vi "SRDG535.panel.vi"(0 "object ref":refnum<vi>, 5 "error in (no error)":errorcluster) -> (19 "error out":errorcluster)   [LabVIEW 2014, in "SRDG535.lvlib"]
doc: "By this VI an ignitron can be monitored and switched. \n\n\"HEATING ON\" and \"WATER ON\" indicate the status (blue: bad tag value, no connection, or internal problems; lightgreen: on; red: off).\n\nThe button switches the electronic of the ignitron, \"SWITCH STATE\" indicates the switch status (blue: bad tag value, no connection, or internal problems; darkgreen: off; lightgreen: on).\n\n\"TRIGGER\" and \"TRIGGER PULSE\" indicate the status of the trigger (blue: bad tag value, no connection, or internal problems; darkgreen: off; lightgreen: on).\n\n\"on since\" indicates at which time the Ignition has been switched on.\n\n\"EXIT\" closes the front panel (GUI), while \"Delete Instance\" disconnects and removes the instance from the PCS.\n\nThis VI has no machine safety relevant logig: there is neither a check of internal conclict nor with other objects. Therefore it must be handled with care and should be operated by well educated operators only. It is forseen exclusively for direct operating and testing of the system. \n\nLicense Agreement for this software:\n\nCopyright (C)\nGesellschaft für Schwerionenforschung, GSI\nPlanckstr. 1\n64291 Darmstadt\nGermany\n\nContact: D.Beck@gsi.de \n\nThis program is free software; you can redistribute it and/or modify it under the terms of the GNU General Public License as published by the Free Software Foundation; either version 2 of the license, or (at your option) any later version.\n\nThis program is distributed in the hope that it will be useful, but WITHOUT ANYW ARRANTY; without even the implied warranty of MERCHANTABILITY or FITNESS FOR A PARTICULAR PURPOSE. See the GNU General License for more details (http://www.gnu.org).\n\nGesellschaft für Schwerionenforschung, GSI\nPlanckstr. 1, 64291 Darmstadt, Germany\nFor all questions and ideas contact: M.Richter@gsi.de, H.Brand@gsi.de or D.Beck@gsi.de.\nLast update: 18-DEC-2002"
uses:
  SRDG535.lvlib
  CS_PHELIX/PH_Basics/PH_StatusHandler/PH_StatusHandler.GUI element.ctl
  SRDG535.Output.ctl
  SRDG535.Channel Output.ctl
  SRDG535.Delay.ctl
  SRDG535.Trigger.ctl
  CS_Core/CSObj/CSObj.lvlib
  CS_PHELIX/PH_Basics/PH_Common/PH_Common.lvlib
  CS_PHELIX/PH_Basics/PH_Class/PH_Class.lvlib
  CS_PHELIX/PH_Basics/PH_PSDBWriter/PH_PSDBWriter.lvlib
  CS_PHELIX/PH_Basics/PH_StatusHandler/PH_StatusHandler.lvlib
panel:
  out "PSDB Status":u32(colorbox)=6618880 caption="PSDB"
  in  "Tab Control":enum32{"Output", "Delay", "Trigger"}(tab)
  out "Output":T1={"CH T0"={"Inversion"=FALSE, "Amplitude (V)"=1.0, "Offset (V)"=0.0, "Mode"=0, "Load"=FALSE}, "CH A"={"Inversion"=FALSE, "Amplitude (V)"=1.0, "Offset (V)"=0.0, "Mode"=0, "Load"=FALSE}, "CH B"={"Inversion"=FALSE, "Amplitude (V)"=1.0, "Offset (V)"=0.0, "Mode"=0, "Load"=FALSE}, "CH AB"={"Inversion"=FALSE, "Amplitude (V)"=1.0, "Offset (V)"=0.0, "Mode"=0, "Load"=FALSE}, "CH C"={"Inversion"=FALSE, "Amplitude (V)"=1.0, "Offset (V)"=0.0, "Mode"=0, "Load"=FALSE}, "CH D"={"Inversion"=FALSE, "Amplitude (V)"=1.0, "Offset (V)"=0.0, "Mode"=0, "Load"=FALSE}, "CH CD"={"Inversion"=FALSE, "Amplitude (V)"=1.0, "Offset (V)"=0.0, "Mode"=0, "Load"=FALSE}} {"CH CD"."Mode" items=["TTL", "NIM", "ECL", "VAR"]; "CH CD"."Offset (V)" min=-3.0 max=4.0 format="%.2f"; "CH CD"."Amplitude (V)" min=-3.0 max=4.0 format="%.2f"; "CH D"."Mode" items=["TTL", "NIM", "ECL", "VAR"]; "CH D"."Offset (V)" min=-3.0 max=4.0 format="%.2f"; "CH D"."Amplitude (V)" min=-3.0 max=4.0 format="%.2f"; "CH C"."Mode" items=["TTL", "NIM", "ECL", "VAR"]; "CH C"."Offset (V)" min=-3.0 max=4.0 format="%.2f"; "CH C"."Amplitude (V)" min=-3.0 max=4.0 format="%.2f"; "CH AB"."Mode" items=["TTL", "NIM", "ECL", "VAR"]; "CH AB"."Offset (V)" min=-3.0 max=4.0 format="%.2f"; "CH AB"."Amplitude (V)" min=-3.0 max=4.0 format="%.2f"; "CH B"."Mode" items=["TTL", "NIM", "ECL", "VAR"]; "CH B"."Offset (V)" min=-3.0 max=4.0 format="%.2f"; "CH B"."Amplitude (V)" min=-3.0 max=4.0 format="%.2f"; "CH A"."Mode" items=["TTL", "NIM", "ECL", "VAR"]; "CH A"."Offset (V)" min=-3.0 max=4.0 format="%.2f"; "CH A"."Amplitude (V)" min=-3.0 max=4.0 format="%.2f"; "CH T0"."Mode" items=["TTL", "NIM", "ECL", "VAR"]; "CH T0"."Offset (V)" min=-3.0 max=4.0 format="%.2f"; "CH T0"."Amplitude (V)" min=-3.0 max=4.0 format="%.2f"}
  out "Delay":T3 {"CH D"."Delay (s)" format="%#_13g"; "CH D"."rel to" scale=0.0..3.0; "CH C"."Delay (s)" format="%#_13g"; "CH C"."rel to" scale=0.0..3.0; "CH B"."Delay (s)" format="%#_13g"; "CH B"."rel to" scale=0.0..3.0; "CH A"."Delay (s)" format="%#_13g"; "CH A"."rel to" scale=0.0..3.0}
  out "Trigger":T4={"trigger"=0, "Impedance"=FALSE, "Slope"=FALSE, "burst count"=2, "external level (V)"=0.0, "Internal/Burst Rate (Hz)"=0.001, "Burst Period"=4} {"Burst Period" min=4 max=32766; "Internal/Burst Rate (Hz)" min=0.001 max=1000000.0 format="%.3f"; "external level (V)" min=-2.56 max=2.56 format="%.2f"; "burst count" min=2 max=32766; "trigger" scale=0.0..4.0}
  out "Device Error":errorcluster
  out "Information":cluster{"GPIB address":string}={"GPIB address"="N/A"}
  out "Status":T5 caption="Enabling State"
  in  "Delete":bool
  in  "Exit":bool
  # "PCS"
  # "3.40"
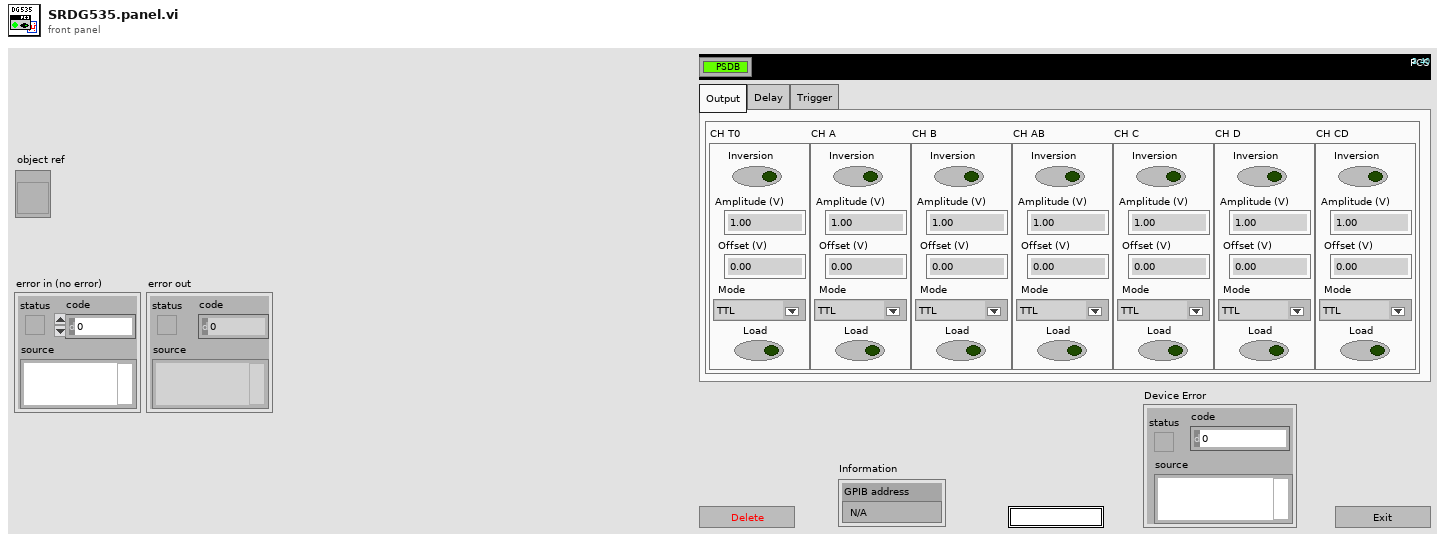
[diagram p1: front panel]
types:
  T1 = typedef "SRDG535.lvlib/SRDG535.Output.ctl" = cluster{"CH T0":T2, "CH A":T2, "CH B":T2, "CH AB":T2, "CH C":T2, "CH D":T2, "CH CD":T2}
  T2 = typedef "SRDG535.lvlib/SRDG535.Channel Output.ctl" = cluster{"Inversion":bool, "Amplitude (V)":dbl, "Offset (V)":dbl, "Mode":i32, "Load":bool}
  T3 = typedef "SRDG535.lvlib/SRDG535.Delay.ctl" = cluster{"CH A":cluster{"rel to":u32, "Delay (s)":dbl}, "CH B":cluster{"rel to":u32, "Delay (s)":dbl}, "CH C":cluster{"rel to":u32, "Delay (s)":dbl}, "CH D":cluster{"rel to":u32, "Delay (s)":dbl}}
  T4 = typedef "SRDG535.lvlib/SRDG535.Trigger.ctl" = cluster{"trigger":u32, "Impedance":bool, "Slope":bool, "burst count":i32, "external level (V)":sgl, "Internal/Burst Rate (Hz)":dbl, "Burst Period":i32}
  T5 = typedef "PH_StatusHandler.lvlib/PH_StatusHandler.GUI element.ctl" = u16
  T6 = typedef "SRDG535.lvlib/SRDG535.i attribute.ctl" = cluster{"GPIB address":string, "Device error":errorcluster, "GUI Refs":cluster{"Delete":refnum<vi>, "Device Error":refnum<vi>, "Information":refnum<vi>, "Output":refnum<vi>, "Delay":refnum<vi>, "Trigger":refnum<vi>}, "Output Settings":T1, "Service ID Rate":i32, "Service IDs Channelinfo":i32[], "Delay Settings":T3, "Trigger Settings":T4}
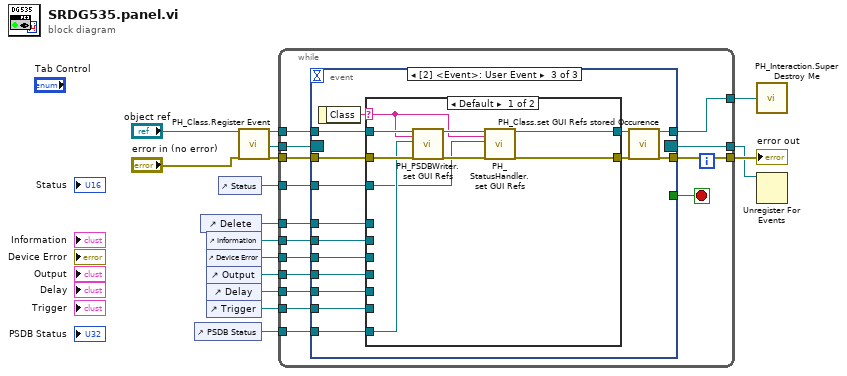
[diagram p0: block diagram]
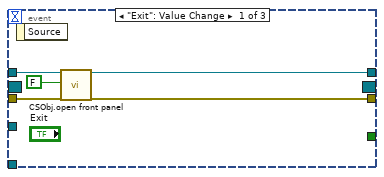
[diagram p2: hidden frame]
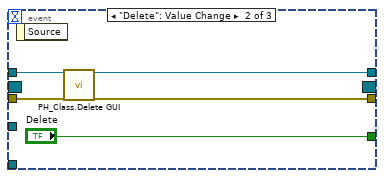
[diagram p3: hidden frame]
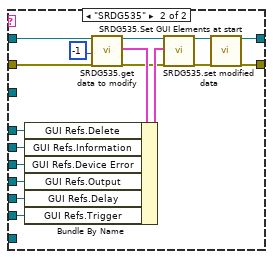
[diagram p4: hidden frame]
diagram:
  n1 = control-ref of="PSDB Status"() -> (w2:refnum<vi>)
  n2 = control-ref of="Delete"() -> (w8:refnum<vi>)
  n3 = control-ref of="Information"() -> (w7:refnum<vi>)
  n4 = control-ref of="Device Error"() -> (w6:refnum<vi>)
  n5 = control-ref of="Output"() -> (w5:refnum<vi>)
  n6 = control-ref of="Delay"() -> (w4:refnum<vi>)
  n7 = control-ref of="Trigger"() -> (w3:refnum<vi>)
  n8 = control-ref of="Status"() -> (w1:refnum<vi>)
  n9 = call "PH_Class.Register Event.vi"("i ref in"="object ref", "error in (no error)"="error in (no error)") -> ("i ref out"=w14:refnum<vi>, "Event Registration Refnum"=w12:refnum<event-registration>, "error out"=w13:errorcluster)  [unwired: 15 in]
  n10 = while {
    tunnel: w14 -> [w28]
    tunnel: [w27] -> w16
    tunnel: w13 -> [w30]
    tunnel: [w29] -> w15
    tunnel: w12 -> [w26]
    tunnel: [w25] -> w11
    tunnel: w8 -> [w24]
    tunnel: w1 -> [w23]
    tunnel: w7 -> [w22]
    tunnel: w6 -> [w21]
    tunnel: w5 -> [w20]
    tunnel: w4 -> [w19]
    tunnel: w3 -> [w18]
    tunnel: w2 -> [w17]
    stop <- w31 stop-if-true
    n11 = event shown="[2] <Event>: User Event" {
      selector: w26 -> [_ _ _]
      dyn-events: [_ _ _] -> w25
      timeout: _ -> [_ _ _]
      tunnel: [_ "Delete" _] -> w31
      tunnel: w28 -> [w36 w40 w54]
      tunnel: w30 -> [w34 w39 w52]
      tunnel: [w33 w38 w55] -> w29
      tunnel: [w32 w37 w56] -> w27
      tunnel: w24 -> [_ _ w50]
      tunnel: w23 -> [_ _ w49]
      tunnel: w22 -> [_ _ w48]
      tunnel: w21 -> [_ _ w47]
      tunnel: w20 -> [_ _ w46]
      tunnel: w19 -> [_ _ w45]
      tunnel: w18 -> [_ _ w44]
      tunnel: w17 -> [_ _ w42]
      event "Exit": Value Change {
        n12 = event-data() -> ()  [unwired: 1 in, 1 out]
        n13 = call "CSObj.open front panel.vi"("i ref in"=w36, "frontPanelOpen"=FALSE ("front panel open"), "error in (no error)"=w34) -> ("i ref out"=w32:refnum<vi>, "error out"=w33:errorcluster)  [unwired: 15 in]
      }
      event "Delete": Value Change {
        n14 = event-data() -> ()  [unwired: 1 in, 1 out]
        n15 = call "PH_Class.Delete GUI.vi"("VI in"=w40, "error in (no error)"=w39) -> ("VI out"=w37:refnum<vi>, "error out"=w38:errorcluster)  [unwired: 16 in]
      }
      event User Event {
        n16 = event-data() -> ("Class"=w43:string)  [unwired: 1 in]
        n17 = case shown="Default" w43 {
          selector: w43 -> [w58 _]
          tunnel: w54 -> [w65 w77]
          tunnel: [w59 w67] -> w53
          tunnel: w52 -> [w64 w76]
          tunnel: [w61 w66] -> w51
          tunnel: w50 -> [_ w75]
          tunnel: w49 -> [w57 _]
          tunnel: w48 -> [_ w74]
          tunnel: w47 -> [_ w73]
          tunnel: w46 -> [_ w72]
          tunnel: w45 -> [_ w71]
          tunnel: w44 -> [_ w70]
          tunnel: w42 -> [w62 _]
          frame Default {
            n18 = call "PH_PSDBWriter.set GUI Refs.vi"("i ref in"=w65, "Class"=w58, "Ref PSDB Status"=w62, "error in"=w64) -> ("i ref out"=w60:refnum<vi>, "error out"=w63:errorcluster)  [unwired: 14 in]
            n19 = call "PH_StatusHandler.set GUI Refs.vi"("i ref in"=w60, "Class"=w58, "GUI Ref"=w57, "error in (no error)"=w63) -> ("i ref out"=w59:refnum<vi>, "error out"=w61:errorcluster)  [unwired: 14 in]
          }
          frame "SRDG535" {
            n20 = call "SRDG535.get data to modify.vi"("i ref in"=w77, "ms timeout (10000)"=-1, "error in (no error)"=w76) -> ("i ref out"=w78:refnum<vi>, "i attribute"=w80:T6, "error out"=w79:errorcluster)  [unwired: 13 in, 1 out]
            n21 = Bundle By Name(cluster=w80, "GUI Refs.Delete"=w75, "GUI Refs.Information"=w74, "GUI Refs.Device Error"=w73, "GUI Refs.Output"=w72, "GUI Refs.Delay"=w71, "GUI Refs.Trigger"=w70) -> (w81:T6)
            n22 = call "SRDG535.set modified data.vi"("i ref in"=w78, "i attribute"=w81, "error in (no error)"=w79) -> ("i ref out"=w69:refnum<vi>, "error out"=w68:errorcluster)  [unwired: 15 in]
            n23 = call "SRDG535.Set GUI Elements at start.vi"("i ref in"=w69, "error in"=w68) -> ("i ref out"=w67:refnum<vi>, "error out"=w66:errorcluster)  [unwired: 16 in]
          }
        }
        n24 = call "PH_Class.set GUI Refs stored Occurence.vi"("i ref in"=w53, "error in (no error)"=w51) -> ("i ref out"=w56:refnum<vi>, "error out"=w55:errorcluster)  [unwired: 16 in]
      }
    }
  }
  "error out" <- w15
  n25 = call "PH_Interaction.Super Destroy Me.vi"("i ref out"=w16) -> ()
  n26 = Unregister For Events(event registration refnum=w11) -> ()  [unwired: 1 in, 1 out]
